vi "PLC_SETTING_VALUES.vi"(8 "error in (no error)":errorcluster, 11 "Modbus Master in":refnum<class "Modbus Master.lvclass">) -> (0 "error out":errorcluster, 3 "Modbus Master out":refnum<class "Modbus Master.lvclass">)   [LabVIEW 2017]
doc: "This vi is used to setting values and reset values"
uses:
  <vilib>/NI/Modbus Library/API/Master/Modbus Master.lvclass
  Global/PLC_to_Auto.vi
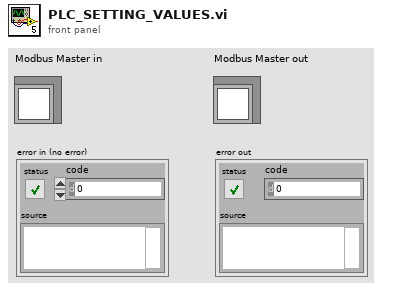
[diagram p1: front panel]
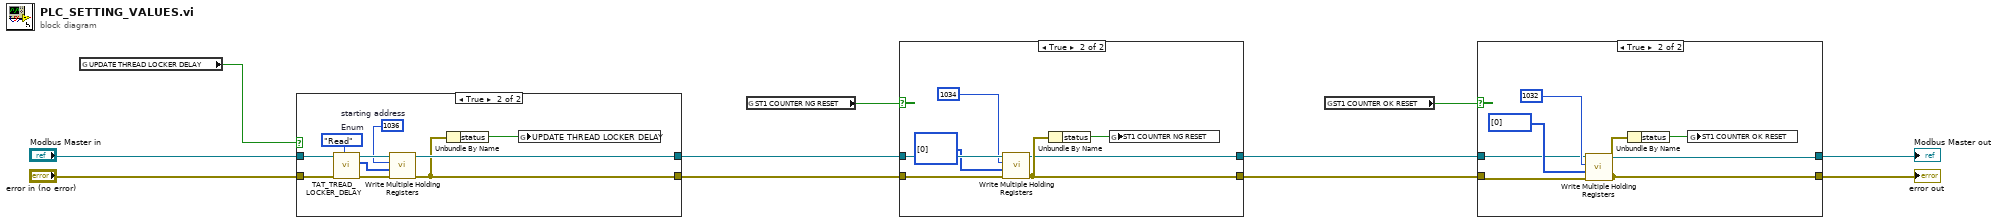
[diagram p0: block diagram]
diagram:
  n1 = global read "PLC_to_Auto.vi" "UPDATE THREAD LOCKER DELAY"() -> (w11:bool)
  n2 = case shown="True" w11 {
    tunnel: [w12 w14] -> w7
    tunnel: "Modbus Master in" -> [w13 w22]
    tunnel: [w13 w21] -> w6
    tunnel: "error in (no error)" -> [w12 w20]
    frame False {
    }
    frame True {
      w18 = enum16{"Read", "Write"}."Read"  # Enum
      w19 = u16 1036  # starting address
      n3 = call "TAT_TREAD_LOCKER_DELAY.vi"("Enum"=w18, "error in (no error)"=w20) -> ("error out"=w16:errorcluster, "Array 2"=w17:u16[])  [unwired: 8 in]
      n4 = call-dynamic "Write Multiple Holding Registers.vi"("error in"=w16, "registers to write"=w17, "starting address"=w19, "Modbus master in"=w22) -> ("error out"=w14:errorcluster, "Modbus master out"=w21:refnum<class "Modbus Master.lvclass">)  [unwired: 6 in]
      n5 = Unbundle By Name(w14) -> ("status"=w15:bool)
      n6 = global write "PLC_to_Auto.vi" "UPDATE THREAD LOCKER DELAY"(w15) -> ()
    }
  }
  n7 = global read "PLC_to_Auto.vi" "ST1 COUNTER NG RESET"() -> (w8:bool)
  n8 = case shown="True" w8 {
    tunnel: [w23 w30] -> w2
    tunnel: w6 -> [w24 w28]
    tunnel: [w24 w27] -> w1
    tunnel: w7 -> [w23 w29]
    frame False {
    }
    frame True {
      n9 = call-dynamic "Write Multiple Holding Registers.vi"("error in"=w29, "registers to write"=i32[] [0], "starting address"=u16 1034, "Modbus master in"=w28) -> ("error out"=w30:errorcluster, "Modbus master out"=w27:refnum<class "Modbus Master.lvclass">)  [unwired: 6 in]
      n10 = Unbundle By Name(w30) -> ("status"=w31:bool)
      n11 = global write "PLC_to_Auto.vi" "ST1 COUNTER NG RESET"(w31) -> ()
    }
  }
  n12 = global read "PLC_to_Auto.vi" "ST1 COUNTER OK RESET"() -> (w5:bool)
  n13 = case shown="True" w5 {
    tunnel: [w32 w36] -> w3
    tunnel: w1 -> [w33 w34]
    tunnel: [w33 w35] -> w4
    tunnel: w2 -> [w32 w37]
    frame False {
    }
    frame True {
      n14 = call-dynamic "Write Multiple Holding Registers.vi"("error in"=w37, "registers to write"=i32[] [0], "starting address"=u16 1032, "Modbus master in"=w34) -> ("error out"=w36:errorcluster, "Modbus master out"=w35:refnum<class "Modbus Master.lvclass">)  [unwired: 6 in]
      n15 = Unbundle By Name(w36) -> ("status"=w40:bool)
      n16 = global write "PLC_to_Auto.vi" "ST1 COUNTER OK RESET"(w40) -> ()
    }
  }
  "error out" <- w3
  "Modbus Master out" <- w4
